vi "Set Domain.vi"(8 "error in (no error)":errorcluster, 10 "domain":variant, 11 "Domain_Evolut_1D in":refnum<class "NI_Domain_Evolut_1D.lvclass">) -> (0 "error out":errorcluster, 3 "Domain_Evolut_1D out":refnum<class "NI_Domain_Evolut_1D.lvclass">)   [LabVIEW 2020, in "NI_PDE.lvlib" / "NI_Domain_Evolut_1D.lvclass"]
uses:
  <vilib>/gmath/pde.llb/DomainClass/Domain_Evolut_1D/NI_Domain_Evolut_1D.lvclass
  <vilib>/gmath/pde.llb/DomainClass/Domain_Evolut_1D/Domain Data.ctl
  <vilib>/gmath/pde.llb/DomainClass/Domain_Evolut_1D/NI_Domain_Evolut_1D.lvclass/NI_Domain_Evolut_1D.ctl
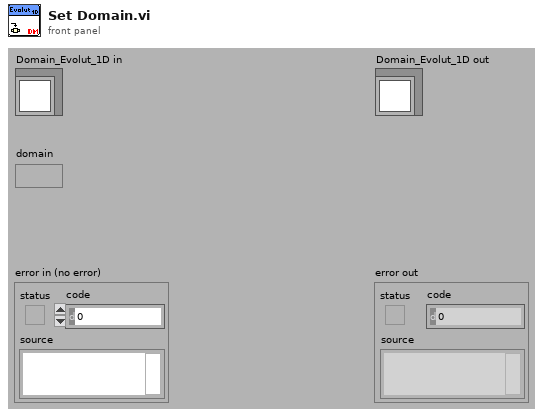
[diagram p1: front panel]
types:
  T1 = typedef "NI_PDE.lvlib/NI_Domain_Evolut_1D.lvclass/Domain Data.ctl" = cluster{"T":cluster{"initial t":dbl, "final t":dbl, "# of t-points":i32}, "X":cluster{"start x":dbl, "end x":dbl, "# of x-points":i32}}
  T2 = cluster{"start x":dbl, "end x":dbl, "# of x-points":i32}
  T3 = cluster{"initial t":dbl, "final t":dbl, "# of t-points":i32}
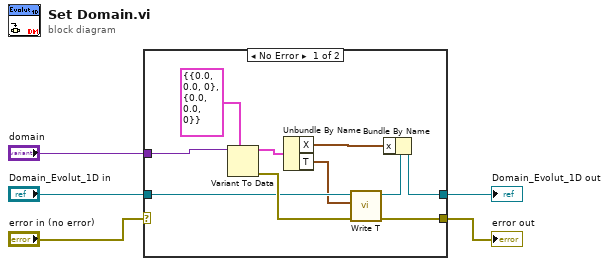
[diagram p0: block diagram]
diagram:
  n1 = case shown="No Error" "error in (no error)" {
    selector: "error in (no error)" -> [_ w17]
    tunnel: "Domain_Evolut_1D in" -> [w12 w16]
    tunnel: [w8 w16] -> w5
    tunnel: [w13 w17] -> w4
    tunnel: "domain" -> [w15 _]
    frame No Error {
      n2 = Variant To Data(type=T1 {"T"={"initial t"=0.0, "final t"=0.0, "# of t-points"=0}, "X"={"start x"=0.0, "end x"=0.0, "# of x-points"=0}} ("domain data"), Variant=w15) -> (data=w11:T1, error out=w14:errorcluster)  [unwired: 1 in]
      n3 = Unbundle By Name(w11) -> ("X"=w7:T2, "T"=w6:T3)
      n4 = call-dynamic "Write T.vi"("error in (no error)"=w14, "t"=w6, "Domain_Evolut.lvclass in"=w12) -> ("error out"=w13:errorcluster, "Domain_Evolut.lvclass out"=w9:refnum<class "NI_Domain_Evolut_1D.lvclass">)  [unwired: 1 in, 6 out]
      n5 = Bundle By Name(cluster=w9, "x"=w7) -> (w8:refnum<class "NI_Domain_Evolut_1D.lvclass">)
    }
    frame Error {
    }
  }
  "Domain_Evolut_1D out" <- w5
  "error out" <- w4
